vi "DSCProgIOC.vi"() -> ()   [LabVIEW 2011]
uses:
  <vilib>/variable/tagger/epicsserver/API/internal/List PVs (By Ref).vi
  <vilib>/variable/tagger/epicsserver/API/internal/Undeploy EPICS Server (By Ref).vi
  <vilib>/variable/tagger/epicsserver/API/NI_EPICS_Server.lvlib
  <vilib>/lvdsc/NI_DSC.lvlib
panel:
  out "error out 3":errorcluster
  out "data out":dbl
  out "error out 2":errorcluster
  out "PVs":string[](array[string])
  out "error out":errorcluster
  in  "stop":bool
  out "EPICS Server URL out":string
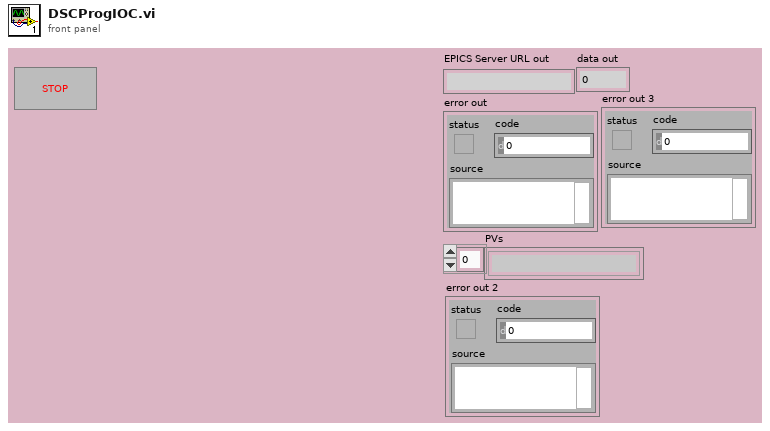
[diagram p1: front panel]
types:
  T1 = enum32{"u32BitField", "bool", "double", "string", "int8", "uint8", "int16", "uint16", "int32", "uint32", "int64", "uint64", "single", "double waveform", "int16 waveform", "array of boolean", "array of int8", "array of uint8", "array of int16", "array of uint16", "array of int32", "array of uint32", "array of int64", "array of uint64", "array of single", "array of double", "array of double waveform", "array of int16 waveform", "array of string", "variant", "timestamp", "fixed point", "custom"}
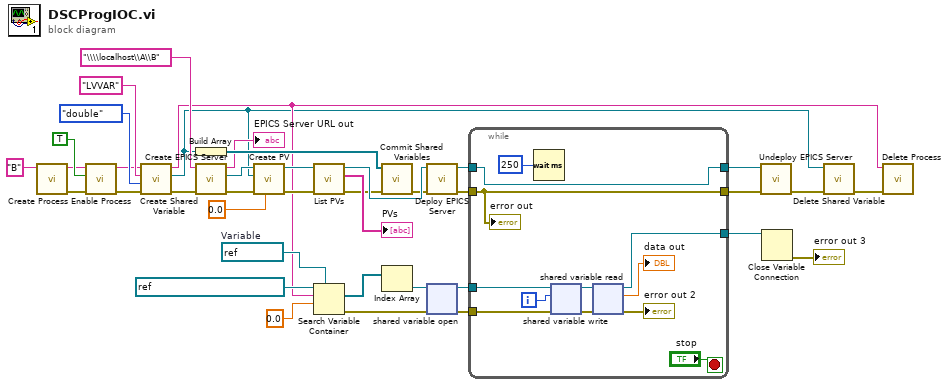
[diagram p0: block diagram]
diagram:
  w20 = refnum<k21> refnum  # Variable
  n1 = call <vilib>:"Create Process.vi"("process name"="B") -> ("error out"=w11:errorcluster, "process name out"=w5:string)  [unwired: 9 in]
  n2 = call <vilib>:"Enable Process.vi"("error in (no error)"=w11, "run?"=TRUE, "process name"=w5) -> ("error out"=w6:errorcluster, "process name out"=w4:string)  [unwired: 7 in]
  n3 = call <vilib>:"Create Shared Variable.vi"("error in (no error)"=w6, "data type"=T1."double", "shared variable name"="LVVAR", "process name"=w4) -> ("error out"=w3:errorcluster, "shared variable"=w1:refnum<k21>, "process name out"=w7:string)  [unwired: 5 in]
  n4 = Build Array(w1) -> (w17:refnum<k21>[])
  n5 = call <vilib>:"Create EPICS Server.vi"("error in (no error)"=w3, "EPICS Server URL in"="\\\\localhost\\A\\B") -> ("error out"=w38:errorcluster, "EPICS Server ref"=w39:refnum<data-value>, "EPICS Server URL out"=→"EPICS Server URL out":string)  [unwired: 7 in]
  n6 = call <vilib>:"Create PV.vi"("data type"=0.0, "error in (no error)"=w38, "variable path"=w1, "EPICS Server ref in"=w39) -> ("error out"=w31:errorcluster, "EPICS Server ref out"=w32:refnum<data-value>)  [unwired: 6 in]
  n7 = call-poly <vilib>:"List PVs.vi"("error in (no error)"=w31, "EPICS Server ref in"=w32) -> ("error out"=w2:errorcluster, "PVs"=→"PVs":string[], "EPICS Server ref out"=w28:refnum<data-value>)  [unwired: 7 in]
  n8 = Search Variable Container(7:w20, 9:0.0, 10:w7, 11:refnum<k21> "ni.var.psp://NDW1032/" ("container refnum in")) -> (0:w15:errorcluster, 2:w24:refnum<k21>[])  [unwired: 2 in, 1 out]
  n9 = call <vilib>:"Commit Shared Variables.vi"("error in (no error)"=w2, "shared variables"=w17) -> ("error out"=w18:errorcluster)  [unwired: 8 in, 1 out]
  n10 = Index Array(array=w24) -> (element=w19:refnum<k21>)  [unwired: 1 in]
  n11 = call <vilib>:"Deploy EPICS Server.vi"("error in (no error)"=w18, "EPICS Server ref in"=w28) -> ("error out"=w27:errorcluster, "EPICS Server ref out"=w35:refnum<data-value>)  [unwired: 8 in]
  n12 = shared-variable-open(w19, w15) -> (w22:refnum<k21>, w14:errorcluster)  [unwired: 1 in]
  n13 = while {
    tunnel: w35 -> [w50]
    tunnel: [w50] -> w34
    tunnel: [w49] -> w33
    tunnel: w27 -> [w49]
    tunnel: w22 -> [w47]
    tunnel: [w44] -> w21
    tunnel: w14 -> [w43]
    i -> [w48]
    stop <- "stop" stop-if-true
    n14 = Wait (ms)(milliseconds to wait=u32 250) -> ()  [unwired: 1 out]
    n15 = shared-variable-write(w47, w43, w48) -> (w46:refnum<k21>, w41:errorcluster)
    n16 = shared-variable-read(w46, w41) -> (w44:refnum<k21>, →"error out 2":errorcluster, →"data out":dbl)  [unwired: 1 out]
    "error out" <- w49
  }
  n17 = call-poly <vilib>:"Undeploy EPICS Server.vi"("error in (no error)"=w33, "EPICS Server ref"=w34) -> ("error out"=w26:errorcluster)  [unwired: 9 in]
  n18 = Close Variable Connection(11:w21) -> (0:→"error out 3":errorcluster)  [unwired: 1 in]
  n19 = call <vilib>:"Delete Shared Variable.vi"("error in (no error)"=w26, "shared variable"=w1) -> ("error out"=w16:errorcluster)  [unwired: 9 in]
  n20 = call <vilib>:"Delete Process.vi"("error in (no error)"=w16, "process name"=w7) -> ()  [unwired: 9 in, 1 out]
